vi "HIOKI PW3390 OPT.vi"(8 "error in (no error)":errorcluster, 11 "VISA Resource":refnum<visa-resource-name>) -> (0 "error out":errorcluster, 2 "OPT":string, 3 "VISA Resource out":refnum<visa-resource-name>)   [LabVIEW 2009]
doc: "Queries the option types attached to the PW3390.\nOutput Items: <CH1 Sensor>, <CH2 Sensor>, <CH3 Sensor>, <CH4 Sensor>"
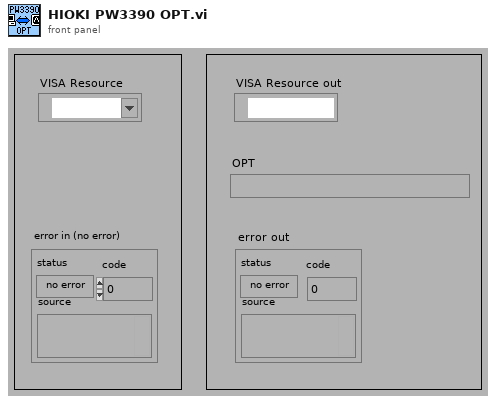
[diagram p1: front panel]
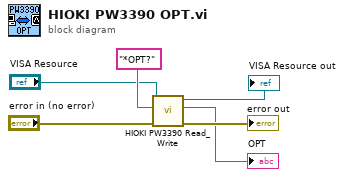
[diagram p0: block diagram]
diagram:
  n1 = call <instrlib>:"HIOKI PW3390 Read_Write.vi"("error in (no error)"="error in (no error)", "data in"="*OPT?", "VISA Resource"="VISA Resource") -> ("error out"=→"error out":errorcluster, "data out"=→"OPT":string, "VISA Resource out"=→"VISA Resource out":refnum<visa-resource-name>)  [unwired: 6 in]
